vi "Write HSDIO.vi"(10 "HSDIO.lvclass":refnum<class "HSDIO.lvclass">, 11 "Experiment in":refnum<class "Experiment.lvclass">) -> (3 "Experiment out":refnum<class "Experiment.lvclass">)   [LabVIEW 2013]
uses:
  Experiment.lvclass
  HSDIO/HSDIO.lvclass
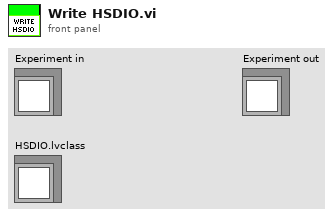
[diagram p1: front panel]
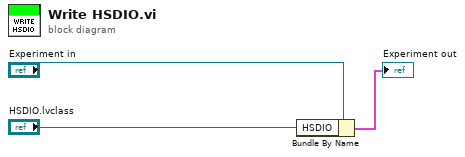
[diagram p0: block diagram]
diagram:
  n1 = Bundle By Name(cluster="Experiment in", "HSDIO"="HSDIO.lvclass") -> (→"Experiment out":cluster{})
